vi "TDMS Open.vi"(7 "Fields In":T1[](array[typedef]), 8 "error in (no error)":errorcluster) -> (0 "error out":errorcluster, 1 "TDMS File Path":path, 2 "Last Run #":i32, 3 "TDMS File Ref":refnum<k34>, 4 "Execution Time (ms)":u32, 5 "Fields Out":T1[](array[typedef]))   [LabVIEW 2011]
uses:
  database/Fields/Field Record.ctl
  database/Fields/Field DataTypes.ctl
  database/Fields/Field NextItem.ctl
  Summitek EXT/OpenG EXT/file/file.llb/Strip Path Extension - String__ogtk.vi
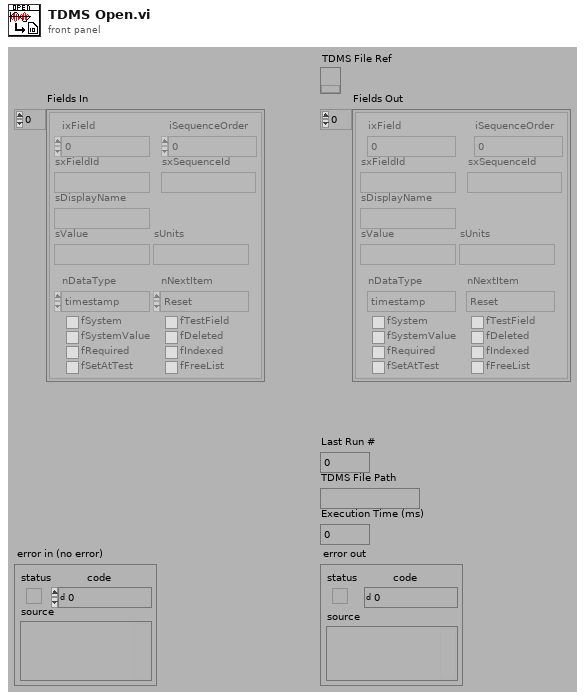
[diagram p1: front panel]
types:
  T1 = typedef "Field Record.ctl" = cluster{"ixField":i32, "iSequenceOrder":i32, "sxFieldId":string, "sxSequenceId":string, "sDisplayName":string, "sValue":string, "sUnits":string, "nDataType":T2, "nNextItem":T3, "fSystem":bool, "fSystemValue":bool, "fRequired":bool, "fSetAtTest":bool, "fTestField":bool, "fDeleted":bool, "fIndexed":bool, "fFreeList":bool}
  T2 = typedef "Field DataTypes.ctl" = enum32{"text", "numeric", "list", "timestamp", "boolean"}
  T3 = typedef "Field NextItem.ctl" = enum32{"Reset", "Retain", "Auto-Increment"}
  T4 = enum16{"open", "open or create", "create or replace", "create", "open (read-only)"}
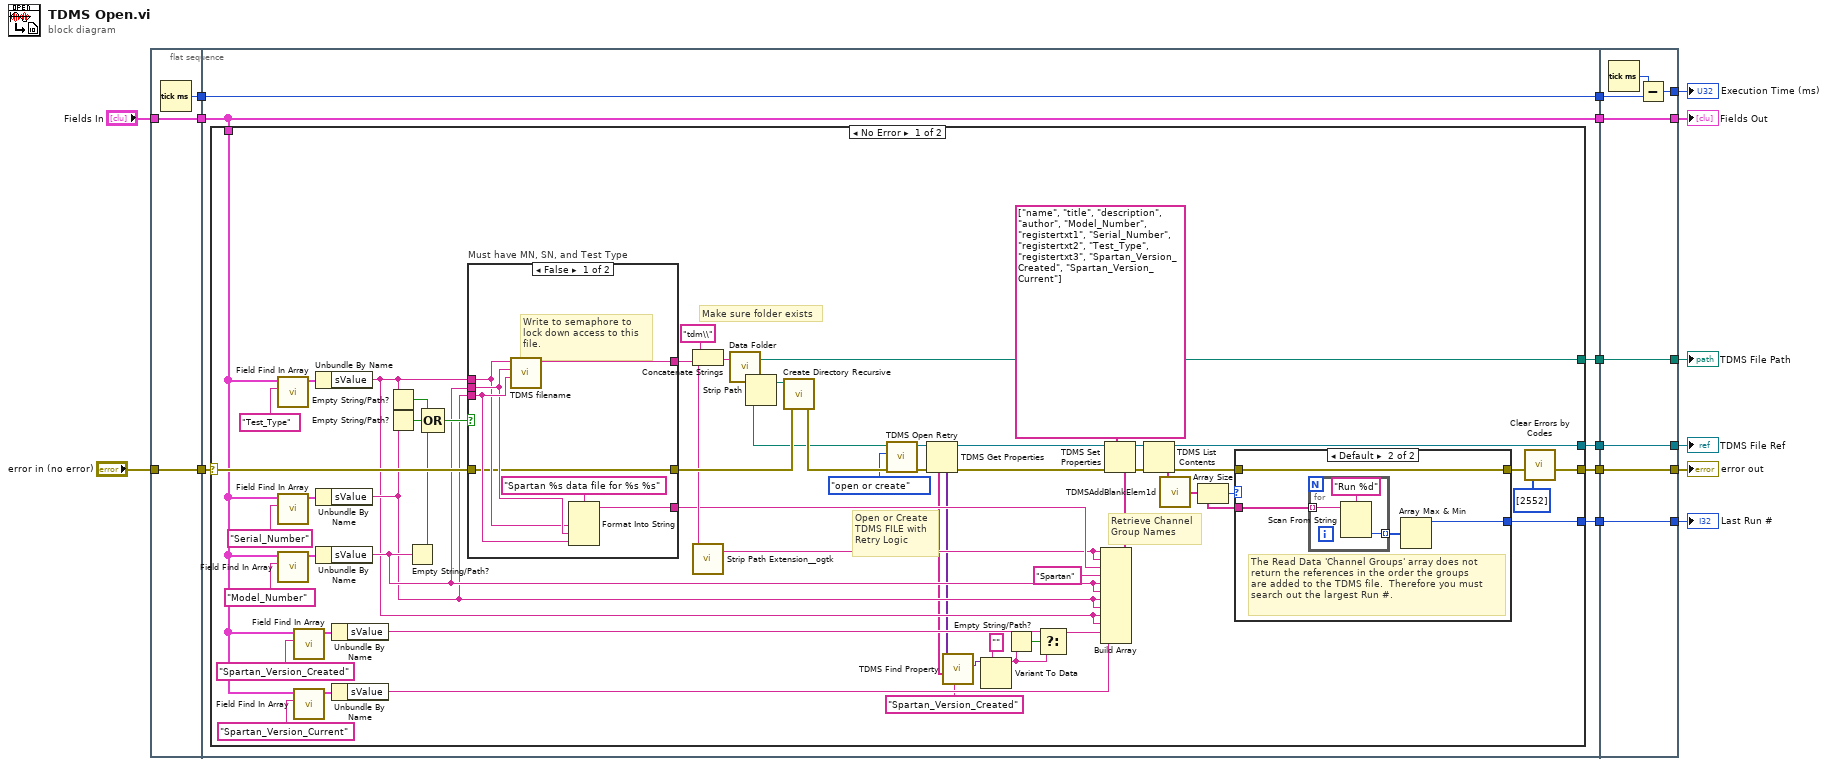
[diagram p0: block diagram]
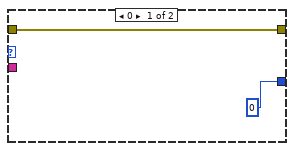
[diagram p2: hidden frame]
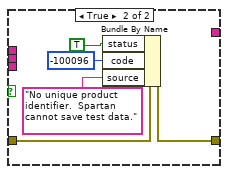
[diagram p3: hidden frame]
diagram:
  n1 = flat-sequence {
    tunnel: [w20] -> w16
    tunnel: [w19] -> w8
    tunnel: "error in (no error)" -> [w19]
    tunnel: [w18] -> w6
    tunnel: "Fields In" -> [w18]
    tunnel: [w27] -> w17
    tunnel: w16 -> [w27]
    tunnel: [w26] -> w13
    tunnel: [w25] -> w11
    tunnel: [w24] -> w10
    tunnel: w8 -> [w23]
    tunnel: w6 -> [w24]
    tunnel: [w22] -> w3
    tunnel: [w21] -> w1
    tunnel: w17 -> [w113]
    tunnel: [w112] -> w15
    tunnel: [w111] -> w14
    tunnel: w13 -> [w111]
    tunnel: [w110] -> w12
    tunnel: w11 -> [w110]
    tunnel: w10 -> [w109]
    tunnel: [w109] -> w9
    tunnel: [w108] -> w4
    tunnel: w3 -> [w108]
    tunnel: [w107] -> w2
    tunnel: w1 -> [w107]
    frame #0 {
      n2 = Tick Count (ms)() -> (millisecond timer value=w20:u32)
    }
    frame #1 {
      n3 = case shown="No Error" w23 {
        selector: w23 -> [w84 w106]
        tunnel: [w78 w106] -> w26
        tunnel: [w79 _] -> w25
        tunnel: w24 -> [w57 _]
        tunnel: [w52 _] -> w22
        tunnel: [w62 _] -> w21
        frame No Error {
          # "Open or Create\nTDMS FILE with\nRetry Logic"
          # "Retrieve Channel\nGroup Names"
          # "Make sure folder exists"
          n4 = call "Field Find In Array.vi"("FieldID or Display Name(\"\")"="Test_Type" ("Field Internal ID"), "Field Array"=w57) -> ("Field"=w75:T1)  [unwired: 1 in, 8 out]
          n5 = call "Field Find In Array.vi"("FieldID or Display Name(\"\")"="Serial_Number" ("Field Internal ID"), "Field Array"=w57) -> ("Field"=w70:T1)  [unwired: 1 in, 8 out]
          n6 = call "Field Find In Array.vi"("FieldID or Display Name(\"\")"="Model_Number" ("Field Internal ID"), "Field Array"=w57) -> ("Field"=w71:T1)  [unwired: 1 in, 8 out]
          n7 = call "Field Find In Array.vi"("FieldID or Display Name(\"\")"="Spartan_Version_Created" ("Field Internal ID"), "Field Array"=w57) -> ("Field"=w58:T1)  [unwired: 1 in, 8 out]
          n8 = call "Field Find In Array.vi"("FieldID or Display Name(\"\")"="Spartan_Version_Current" ("Field Internal ID"), "Field Array"=w57) -> ("Field"=w59:T1)  [unwired: 1 in, 8 out]
          n9 = Unbundle By Name(w75) -> ("sValue"=w54:string)
          n10 = Unbundle By Name(w70) -> ("sValue"=w63:string)
          n11 = Unbundle By Name(w71) -> ("sValue"=w64:string)
          n12 = Unbundle By Name(w58) -> ("sValue"=w55:string)
          n13 = Unbundle By Name(w59) -> ("sValue"=w56:string)
          n14 = Empty String/Path?(string/path=w54) -> (empty?=w76:bool)
          n15 = Empty String/Path?(string/path=w63) -> (empty?=w77:bool)
          n16 = Empty String/Path?(string/path=w64) -> (empty?=w68:bool)
          n17 = Compound Arithmetic op=OR(w76, w77, w68) -> (w69:bool)
          n18 = case "Must have MN, SN, and Test Type" shown="False" w69 {
            tunnel: [w95 _] -> w67
            tunnel: [w100 _] -> w66
            tunnel: w63 -> [w99 _]
            tunnel: w54 -> [w96 _]
            tunnel: w64 -> [w98 _]
            tunnel: w84 -> [w94 w102]
            tunnel: [w94 w101] -> w82
            frame False {
              # "Write to semaphore to\nlock down access to this\nfile."
              n19 = call "TDMS filename.vi"("Serial Number"=w99, "Model Number"=w98, "Test Type"=w96) -> ("Filename"=w95:string)  [unwired: 8 out]
              n20 = Format Into String(format string="Spartan %s data file for %s %s", w96, w98, w99) -> (resulting string=w100:string)  [unwired: 2 in, 1 out]
            }
            frame True {
              n21 = Bundle By Name(cluster=w102, "status"=TRUE, "code"=-100096, "source"="No unique product identifier.  Spartan cannot save test data.") -> (w101:errorcluster)
            }
          }
          n22 = Concatenate Strings("tdm\\", w67) -> (w80:string)
          n23 = call-poly "Strip Path Extension__ogtk.vi"("path"=w67) -> ("root"=w65:string)  [unwired: 1 out]
          n24 = call "Data Folder.vi"("Relative Path (\"\" - Folder)"=w80) -> ("Data Folder"=w52:path)  [unwired: 2 in]
          n25 = Strip Path(path=w52) -> (stripped path=w83:path)  [unwired: 1 out]
          n26 = call <vilib>:"Create Directory Recursive.vi"("error in (no error)"=w82, "directory"=w83) -> ("error out"=w53:errorcluster)  [unwired: 1 in, 4 out]
          n27 = call "TDMS Open Retry.vi"("error in (no error)"=w53, "Operation (0:open)"=T4."open or create" ("operation (0:open)"), "Path"=w52) -> ("error out"=w29:errorcluster, "TDMS File Ref"=w28:refnum<k34>)  [unwired: 1 in, 6 out]
          n28 = TDMS Get Properties(8:w29, 11:w28) -> (0:w41:errorcluster, 3:w40:refnum<k34>, 4:w38:variant[], 6:w37:string[])  [unwired: 6 out]
          n29 = call "TDMS Find Property.vi"("Property Name"="Spartan_Version_Created" ("element"), "Property Names"=w37, "Property Values"=w38) -> ("Property Value"=w36:variant)  [unwired: 5 out]
          n30 = Variant To Data(type="" ("format string"), Variant=w36) -> (data=w33:string)  [unwired: 1 in, 1 out]
          n31 = Empty String/Path?(string/path=w33) -> (empty?=w34:bool)
          n32 = Select(t=w55, s=w34, f=w33) -> (s? t:f=w32:string)
          n33 = Build Array(w65, w65, w66, "Spartan" ("format string"), w64, w64, w63, w63, w54, w54, w32, w56) -> (w50:string[])
          n34 = TDMS Set Properties(5:w50, 7:string[] ["name", "title", "description", "author", "Model_Number", "registertxt1", "Serial_Number", "registertxt2", "Test_Type", "registertxt3", "Spartan_Version_Created", "Spartan_Version_Current"], 8:w41, 11:w40) -> (0:w42:errorcluster, 3:w49:refnum<k34>)  [unwired: 4 out]
          n35 = TDMS List Contents(4:w42, 7:w49) -> (0:w48:errorcluster, 2:w31:string[], 3:w62:refnum<k34>)  [unwired: 2 out]
          n36 = call <vilib>:"TDMSAddBlankElem1d.vi"("input string array"=w31) -> ("output string array with blank element at the beginning"=w47:string[])
          n37 = Array Size(array=w47) -> (size(s)=w51:i32)
          n38 = case shown="Default" w51 {
            tunnel: w47 -> [_ w90]
            tunnel: w48 -> [w85 w87]
            tunnel: [w85 w87] -> w43
            tunnel: [0 w88] -> w79
            frame 0 {
            }
            frame Default {
              # "The Read Data 'Channel Groups' array does not\nreturn the references in the order the groups\nare added to the TDMS file.  Therefore you must\nsearch out the largest Run #."
              n39 = for {
                tunnel: w90 -> [w91] mode=indexing
                tunnel: [w92] -> w89 mode=indexing
                n40 = Scan From String(format string="Run %d", input string=w91) -> (output 1=w92:i32)  [unwired: 2 in, 4 out]
              }
              n41 = Array Max & Min(array=w89) -> (max value=w88:i32)  [unwired: 3 out]
            }
          }
          n42 = call "Clear Errors by Codes.vi"("Error Codes\nto Clear (Empty)"=i32[] [2552] ("Error Codes\nto Clear (Empty)"), "error in (no error)"=w43) -> ("error out"=w78:errorcluster)  [unwired: 5 out]
        }
        frame Error {
        }
      }
    }
    frame #2 {
      n43 = Tick Count (ms)() -> (millisecond timer value=w114:u32)
      n44 = Subtract(x=w114, y=w113) -> (x-y=w112:u32)
    }
  }
  "Execution Time (ms)" <- w15
  "Last Run #" <- w12
  "error out" <- w14
  "Fields Out" <- w9
  "TDMS File Path" <- w4
  "TDMS File Ref" <- w2
